vi "Recieve command.vi"(0 "reference in":refnum<class "CR slave.lvclass">, 11 "error in (no error)":errorcluster, 13 "timeout ms (100)":i32=100) -> (4 "reference out":refnum<class "CR slave.lvclass">, 6 "message":string, 8 "parameters":string, 10 "data":variant, 14 "timed out?":bool, 15 "error out":errorcluster)   [LabVIEW 2019, in "CommandResponse communication.lvlib" / "CR slave.lvclass"]
doc: "Recives command as message + variant data"
uses:
  CR slave.lvclass
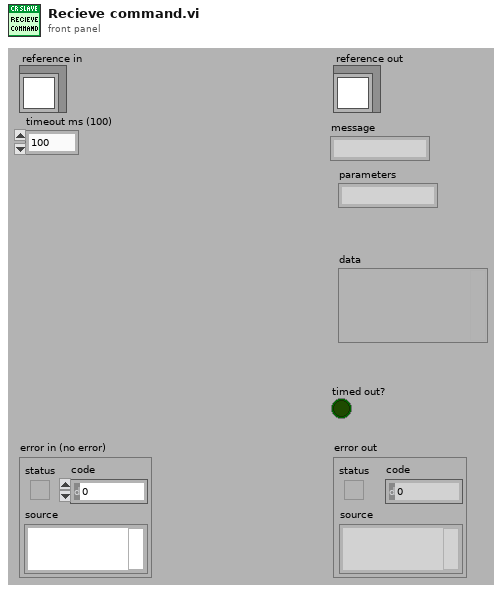
[diagram p1: front panel]
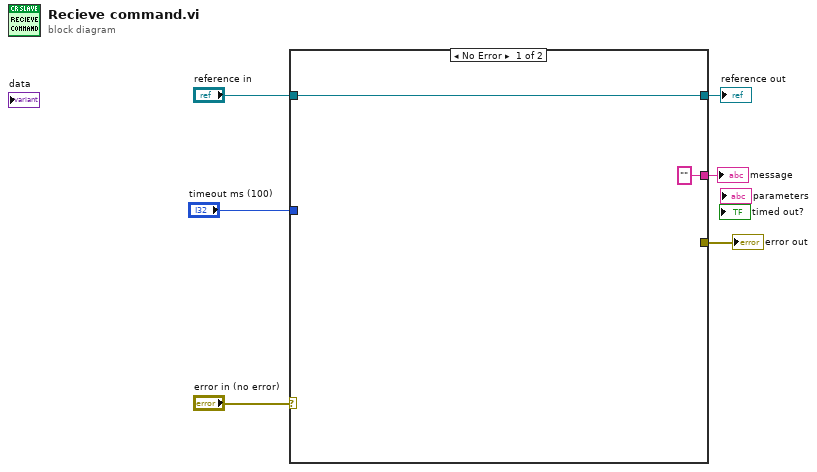
[diagram p0: block diagram]
diagram:
  n1 = case shown="No Error" "error in (no error)" {
    selector: "error in (no error)" -> [_ w10]
    tunnel: [_ w10] -> w5
    tunnel: [w8 w9] -> w3
    tunnel: "reference in" -> [w8 w9]
    tunnel: "timeout ms (100)" -> [_ _]
    tunnel: ["" ("message") _] -> w1
    frame No Error {
    }
    frame Error {
    }
  }
  "error out" <- w5
  "reference out" <- w3
  "message" <- w1
